vi "SetVIInformation.vi"() -> ()   [LabVIEW 2018]
uses:
  Ctr/Cmd.ctl
  Ctr/VIData.ctl
panel:
  in  "VIList":string(combo)
  in  "Exit":bool
  in  "Save":bool
  in  "VI Info":i32(listbox)
  in  "Load":bool
  in  "路径":path
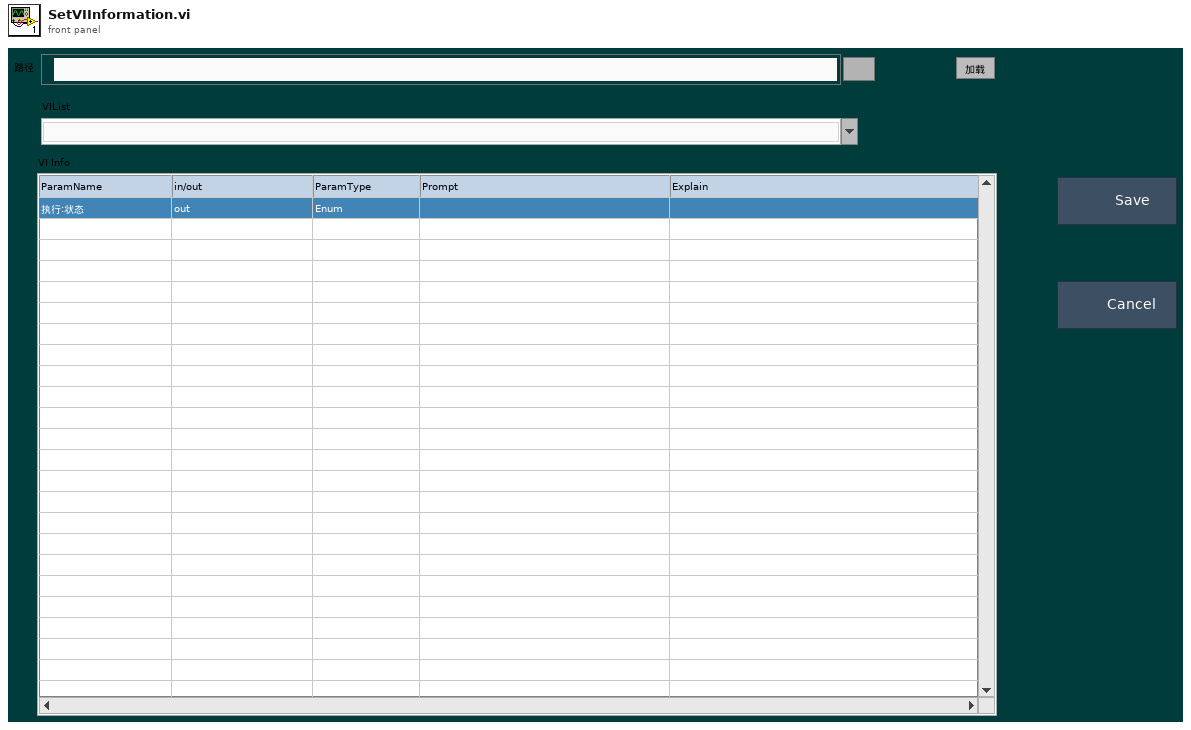
[diagram p1: front panel]
types:
  T1 = typedef "VIData.ctl" = cluster{"VIpath":string, "error":errorcluster}
  T2 = typedef "Cmd.ctl" = enum32{"Idle", "Initial", "SaveFile", "LoadFile", "Error", "Warning", "Exit", "ParseVI", "SaveVI"}
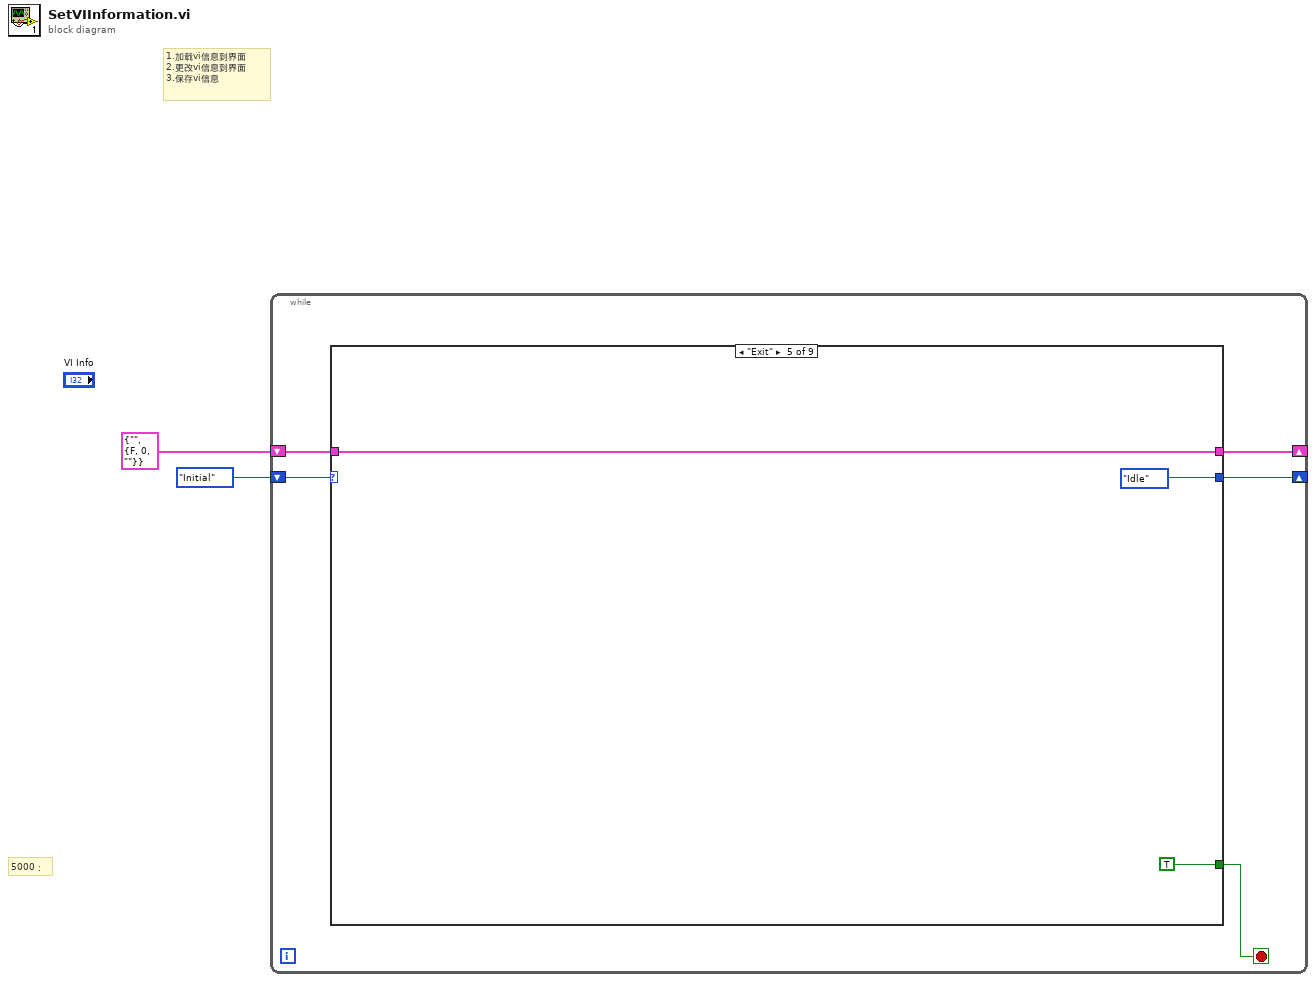
[diagram p0: block diagram]
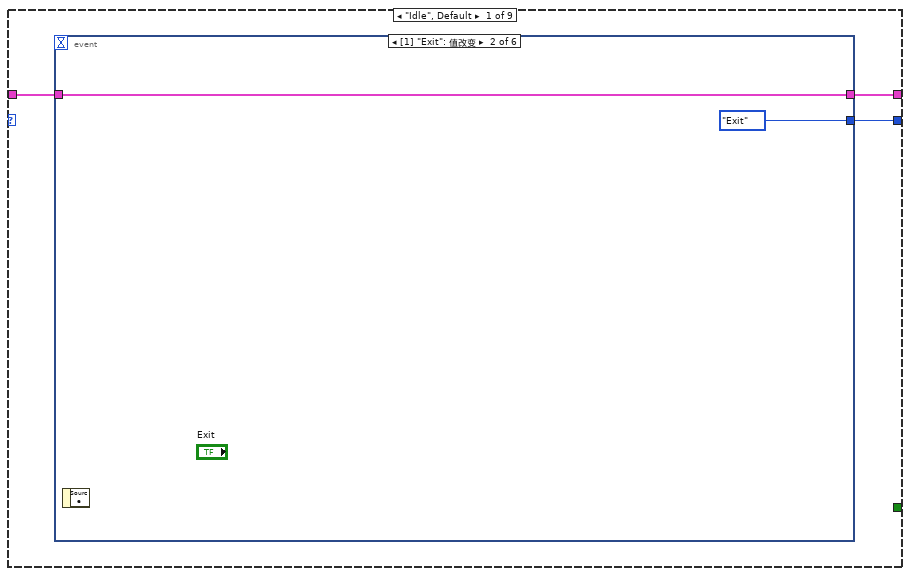
[diagram p2: hidden frame]
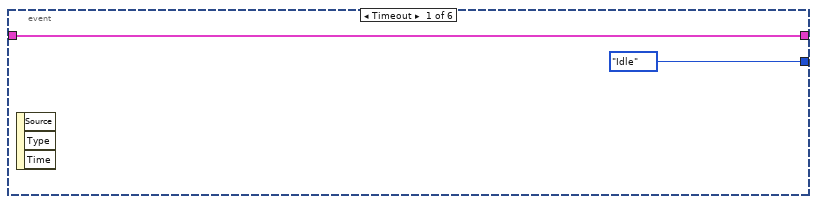
[diagram p3: hidden frame]
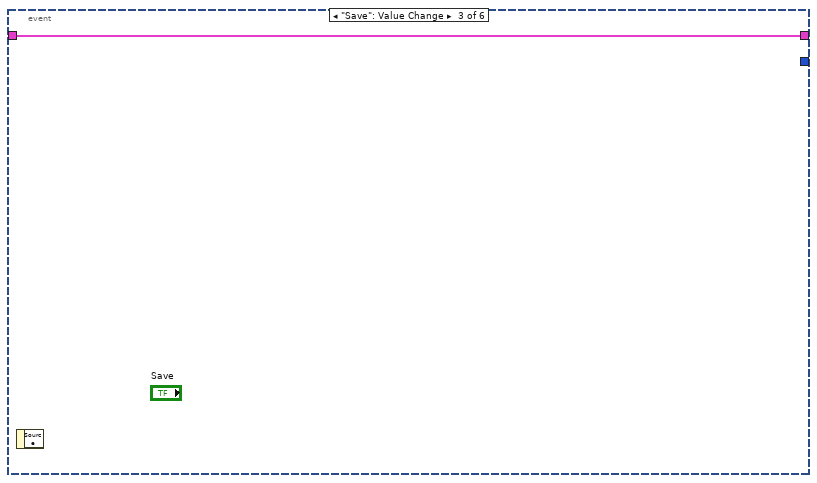
[diagram p4: hidden frame]
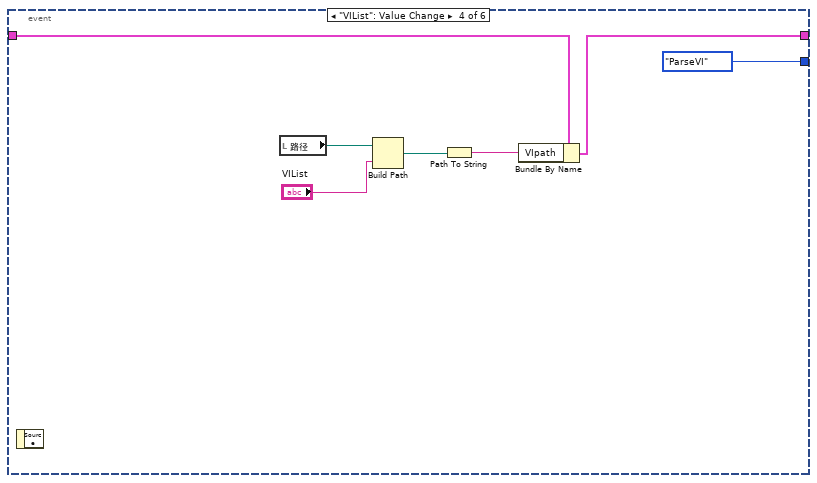
[diagram p5: hidden frame]
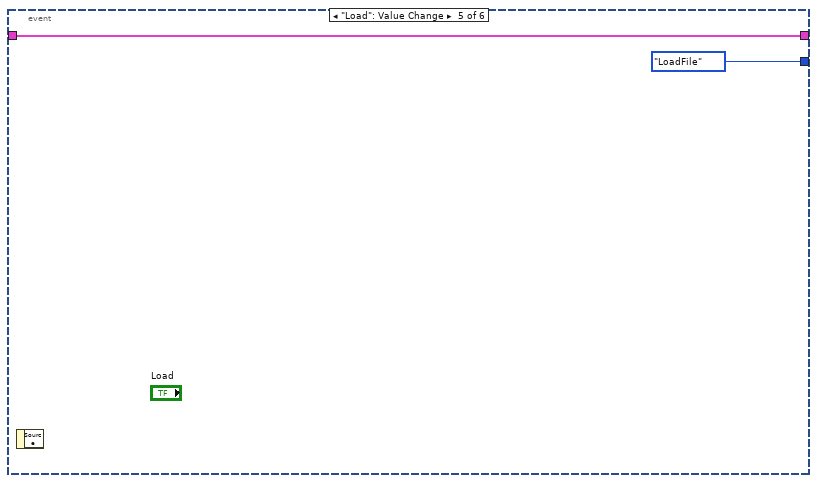
[diagram p6: hidden frame]
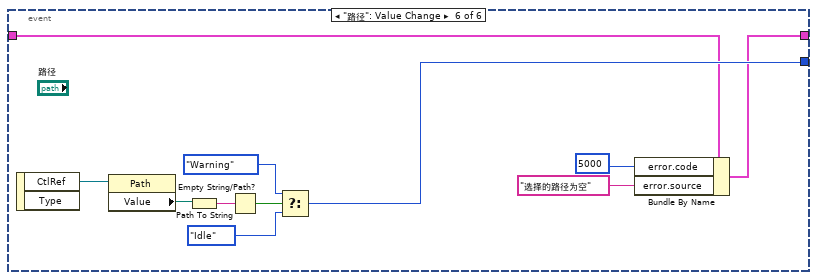
[diagram p7: hidden frame]
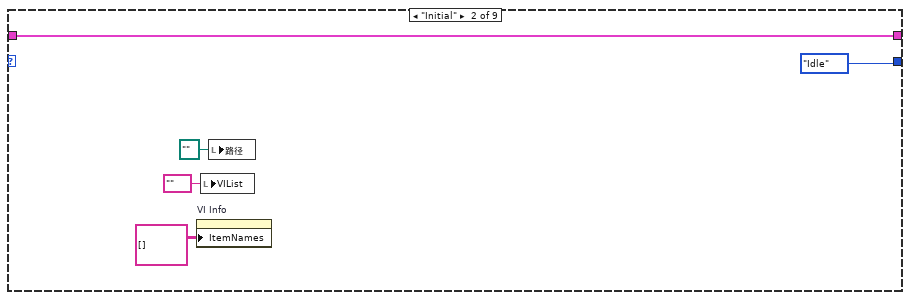
[diagram p8: hidden frame]
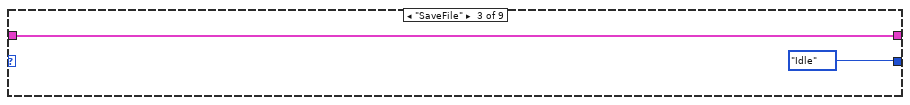
[diagram p9: hidden frame]
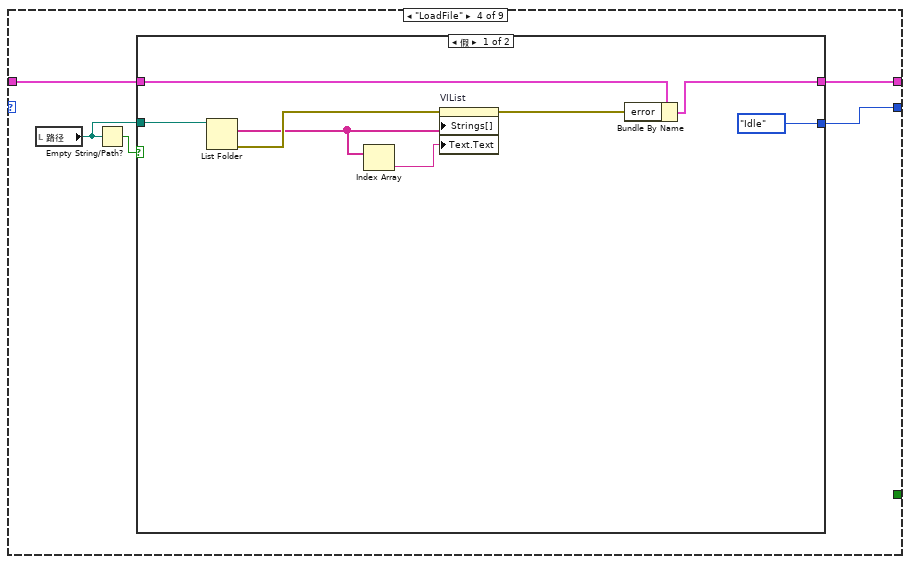
[diagram p10: hidden frame]
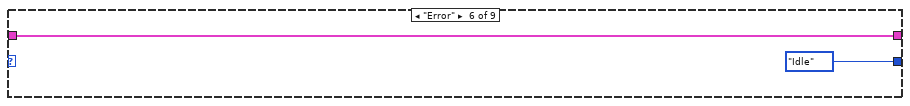
[diagram p12: hidden frame]
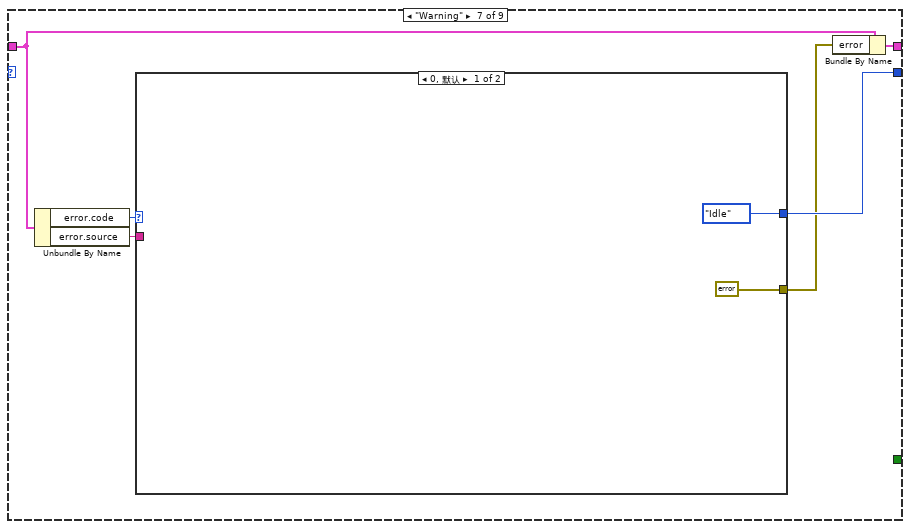
[diagram p13: hidden frame]
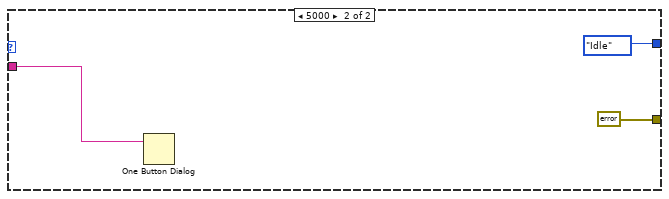
[diagram p14: hidden frame]
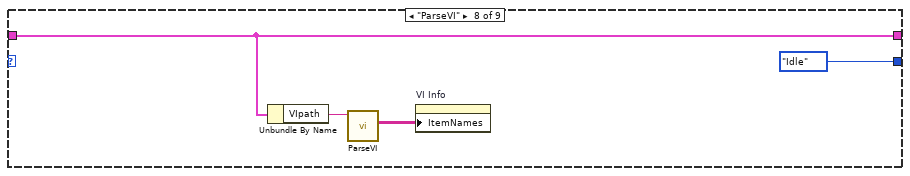
[diagram p15: hidden frame]
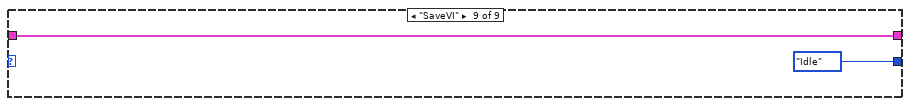
[diagram p16: hidden frame]
diagram:
  # "5000："
  # "1.加载vi信息到界面\n2.更改vi信息到界面\n3.保存vi信息"
  n1 = while {
    shift-right: [w5] -> _
    shift-left: Cmd."Initial" -> [w7]
    shift-right: [w4] -> _
    shift-left: T1 {"VIpath"="", "error"={"status"=FALSE, "code"=0, "source"=""}} ("VIData") -> [w3]
    stop <- w6 stop-if-true
    n2 = case shown="\"Exit\"" w7 {
      tunnel: [_ _ _ _ TRUE _ _ _ _] -> w6
      tunnel: [w10 Cmd."Idle" ("Cmd") Cmd."Idle" ("Cmd") w45 Cmd."Idle" ("Cmd") Cmd."Idle" ("Cmd") w65 Cmd."Idle" ("Cmd") Cmd."Idle" ("Cmd")] -> w5
      tunnel: [w9 w36 w41 w43 w57 w60 w63 w74 w77] -> w4
      tunnel: w3 -> [w8 w36 w41 w44 w57 w60 w64 w74 w77]
      frame "Idle", Default {
        n3 = event shown="[1] \"Exit\": 值改变" {
          selector: _ -> [_ _ _ _ _ _]
          dyn-events: _ -> [_ _ _ _ _ _]
          timeout: _ -> [_ _ _ _ _ _]
          tunnel: [Cmd."Idle" ("Cmd") Cmd."Exit" ("Cmd") _ Cmd."ParseVI" ("Cmd") Cmd."LoadFile" ("Cmd") w29] -> w10
          tunnel: [w11 w14 w15 w18 w23 w28] -> w9
          tunnel: w8 -> [w11 w14 w15 w19 w23 w27]
          event Timeout {
            n4 = event-data() -> ()  [unwired: 1 in, 3 out]
          }
          event "Exit": Value Change {
            n5 = event-data() -> ()  [unwired: 1 in, 1 out]
          }
          event "Save": Value Change {
            n6 = event-data() -> ()  [unwired: 1 in, 1 out]
          }
          event "VIList": Value Change {
            n7 = event-data() -> ()  [unwired: 1 in, 1 out]
            n8 = local read "路径"() -> (w20:path)
            n9 = Build Path(base path=w20, name or relative path="VIList") -> (appended path=w17:path)
            n10 = Path To String(path=w17) -> (string=w16:string)
            n11 = Bundle By Name(cluster=w19, "VIpath"=w16) -> (w18:T1)
          }
          event "Load": Value Change {
            n12 = event-data() -> ()  [unwired: 1 in, 1 out]
          }
          event "路径": Value Change {
            n13 = event-data() -> ("CtlRef"=w35:refnum<vi>)  [unwired: 1 in, 1 out]
            n14 = property class="Path"(reference=w35) -> ("Value"=w34:path)  [unwired: 1 in, 2 out]
            n15 = Path To String(path=w34) -> (string=w33:string)
            n16 = Empty String/Path?(string/path=w33) -> (empty?=w32:bool)
            n17 = Select(t=Cmd."Warning", s=w32, f=Cmd."Idle" ("Cmd")) -> (s? t:f=w29:T2)
            n18 = Bundle By Name(cluster=w27, "error.code"=5000 ("code"), "error.source"="选择的路径为空" ("source")) -> (w28:T1)
          }
        }
      }
      frame "Initial" {
        n19 = property on="VI Info" class="MCListbox (严格)"("ItemNames"=string[][] [] ("项名")) -> ()  [unwired: 2 in, 2 out]
        n20 = local write "VIList"("" ("VIList")) -> ()
        n21 = local write "路径"(path "" ("路径")) -> ()
      }
      frame "SaveFile" {
      }
      frame "LoadFile" {
        n22 = local read "路径"() -> (w46:path)
        n23 = Empty String/Path?(string/path=w46) -> (empty?=w47:bool)
        n24 = case shown="假" w47 {
          tunnel: w46 -> [w55 _]
          tunnel: [Cmd."Idle" ("Cmd") _] -> w45
          tunnel: w44 -> [w50 w56]
          tunnel: [w48 w56] -> w43
          frame False {
            n25 = List Folder(path=w55) -> (filenames=w53:string[], error out=w54:errorcluster)  [unwired: 3 in, 2 out]
            n26 = Index Array(array=w53) -> (element=w52:string)  [unwired: 1 in]
            n27 = property on="VIList" class="CmbBox"(error in=w54, "Strings[]"=w53, "Text.Text"=w52) -> (error out=w49:errorcluster)  [unwired: 1 in, 1 out]
            n28 = Bundle By Name(cluster=w50, "error"=w49) -> (w48:T1)
          }
          frame True {
          }
        }
      }
      frame "Exit" {
      }
      frame "Error" {
      }
      frame "Warning" {
        n29 = Unbundle By Name(w64) -> ("error.code"=w67:i32, "error.source"=w66:string)
        n30 = case shown="0, 默认" w67 {
          tunnel: w66 -> [_ w72]
          tunnel: [Cmd."Idle" ("Cmd") Cmd."Idle" ("Cmd")] -> w65
          tunnel: [errorcluster {"status"=FALSE, "code"=0, "source"=""} ("错误常量") errorcluster {"status"=FALSE, "code"=0, "source"=""} ("错误常量")] -> w62
          frame 0, Default {
          }
          frame 5000 {
            n31 = One Button Dialog(message=w72) -> ()  [unwired: 1 in, 1 out]
          }
        }
        n32 = Bundle By Name(cluster=w64, "error"=w62) -> (w63:T1)
      }
      frame "ParseVI" {
        n33 = Unbundle By Name(w74) -> ("VIpath"=w73:string)
        n34 = call "ParseVI.vi"("VIPath"=w73) -> ("数组"=w75:string[][])  [unwired: 9 in, 1 out]
        n35 = property on="VI Info" class="MCListbox (严格)"("ItemNames"=w75) -> ()  [unwired: 2 in, 2 out]
      }
      frame "SaveVI" {
      }
    }
  }
